vi "Detect QR Code (Greyscale).vi"(8 "error in (no error)":errorcluster, 10 "Greyscale Image":T4, 11 "QR Code Detector in":refnum<class "QR Code Detector.lvclass">) -> (0 "error out":errorcluster, 2 "Detections":T1[](array[typedef]), 3 "QR Code Detector (Duplicate)":refnum<class "QR Code Detector.lvclass">)   [LabVIEW 2020, in "g_ar_toolkit.feature_detection.lvlib" / "QR Code Detector.lvclass"]
uses:
  QR Code Detector.lvclass
  g_ar_toolkit.image/Greyscale Image.ctl
  Detection.ctl
  Detection Region.ctl
  g_ar_toolkit.common/Image Point (Float).ctl
  QR Code Detector.lvclass/QR Code Detector.ctl
  de44e2b3-a41c-416e-9770-09f180cbffa1.vi
  g_ar_toolkit.common/Module Path.vi
  <vilib>/Utility/error.llb/Error Cluster From Error Code.vi
  g_ar_toolkit.common/g_ar_toolkit.common.lvlib
  g_ar_toolkit.image/g_ar_toolkit.image.lvlib
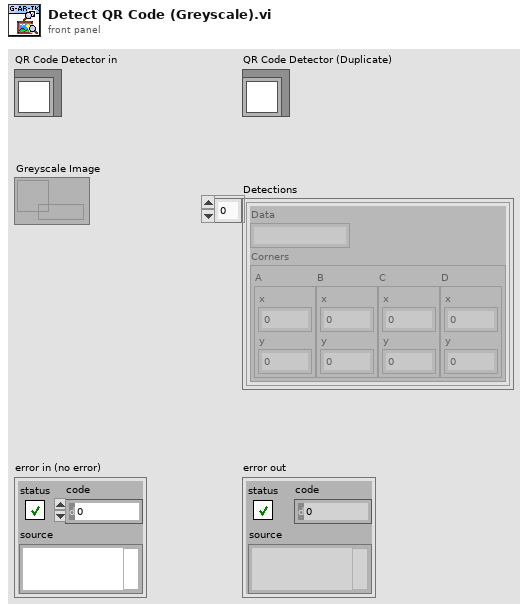
[diagram p1: front panel]
types:
  T1 = typedef "g_ar_toolkit.feature_detection.lvlib/QR Code Detector.lvclass/Detection.ctl" = cluster{"Data":string, "Corners":T2}
  T2 = typedef "g_ar_toolkit.feature_detection.lvlib/QR Code Detector.lvclass/Detection Region.ctl" = cluster{"A":T3, "B":T3, "C":T3, "D":T3}
  T3 = typedef "g_ar_toolkit.common.lvlib/Image Point (Float).ctl" = cluster{"x":dbl, "y":dbl}
  T4 = typedef "g_ar_toolkit.image.lvlib/Greyscale Image.ctl" = refnum<data-value>
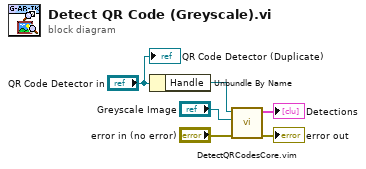
[diagram p0: block diagram]
diagram:
  n1 = Unbundle By Name("QR Code Detector in") -> ("Handle"=w1:refnum<data-value>)
  n2 = call "DetectQRCodesCore.vim"("error in (no error)"="error in (no error)", "Greyscale Image"="Greyscale Image", "Handle"=w1) -> ("error out"=→"error out":errorcluster, "Detections"=→"Detections":T1[])  [unwired: 7 in]
  "QR Code Detector (Duplicate)" <- "QR Code Detector in"
